vi "Test Ignore Private Methods.vi"(11 "Test Case In":refnum<class "Parameterized Test Case Test.lvclass">) -> (0 "error out":errorcluster, 3 "Test Case Out":refnum<class "Parameterized Test Case Test.lvclass">)   [LabVIEW 2020, in "Parameterized Test Case Test.lvclass"]
uses:
  Parameterized Test Case Test.lvclass
  C:/Program Files/National Instruments/LabVIEW 2024/vi.lib/Astemes/LUnit/Test Case.lvclass
  <vilib>/Astemes/LUnit/Test Case.lvclass/Test Case.ctl
  95d5dabd-fcff-41b2-bd37-e613ff77b571.vi
  <vilib>/Astemes/LUnit/Palette/Fail If.vi
  <vilib>/Astemes/LUnit/Core/LUnit Test Case/Private/Append Pass Result.vi
  <vilib>/Astemes/LUnit/Core/LUnit Test Case/Private/Append Fail Result.vi
  <vilib>/Astemes/LUnit/Core/LUnit Test Case/Private/Run In UI.vi
  <vilib>/Utility/error.llb/Clear Errors.vi
  source/Parameterized Test Case/Parameterized Test Case.lvclass
  <vilib>/Astemes/LUnit/Test Suite.lvclass
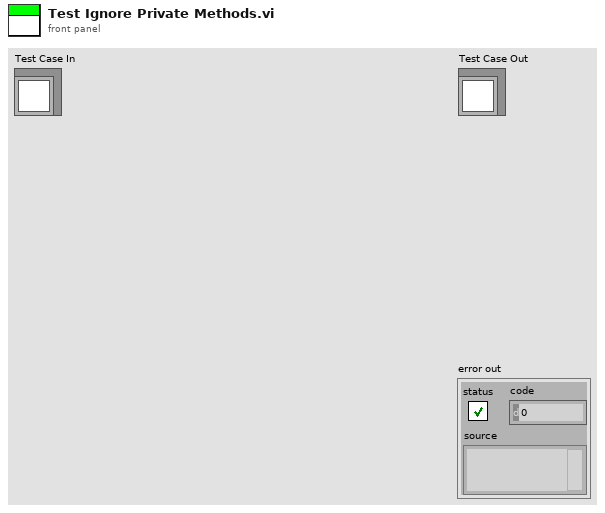
[diagram p1: front panel]
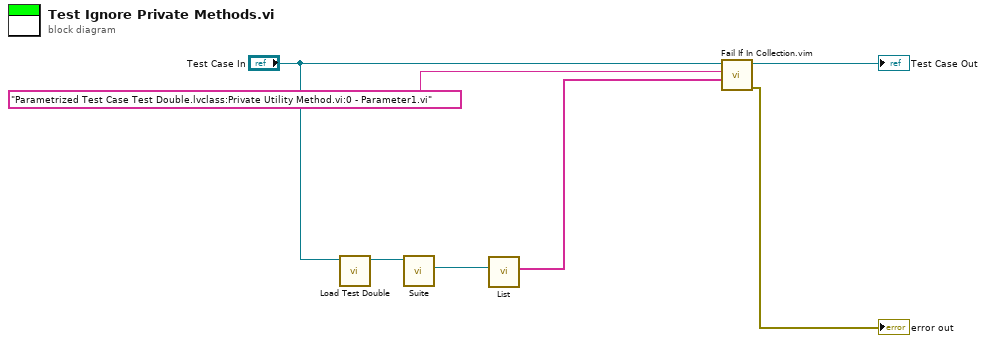
[diagram p0: block diagram]
diagram:
  n1 = call "Load Test Double.vi"("Parameterized Test Case Test in"="Test Case In") -> ("Parameterized Test Case out"=w2:refnum<class "Parameterized Test Case.lvclass">)  [unwired: 9 in, 1 out]
  n2 = call-dynamic "Suite.vi"("Parameterized Test Case In"=w2) -> ("LUnit Test Suite Out"=w4:refnum<class "Test Suite.lvclass">)  [unwired: 8 in, 2 out]
  n3 = call <vilib>:"List.vi"("LUnit Test Suite In"=w4) -> ("List of Runnables"=w3:string[])  [unwired: 9 in, 1 out]
  n4 = call "Fail If In Collection.vim"("Collection"=w3, "Element"="Parametrized Test Case Test Double.lvclass:Private Utility Method.vi:0 - Parameter1.vi" ("String"), "LUnit Test Case In"="Test Case In") -> ("error out"=→"error out":errorcluster, "LUnit Test Case Out"=→"Test Case Out":refnum<class "Parameterized Test Case Test.lvclass">)  [unwired: 7 in]
